vi "TSM Digital Close Sessions.vi"(0 "TSM context":T1) -> (15 "error out":errorcluster)   [LabVIEW 2019]
doc: "Use this VI to reset and close all sessions for all NI-Digital Pattern instruments in the Semiconductor Module Context."
uses:
  <vilib>/NI_TestStand_SemiconductorModule/NI_TestStand_Semiconductor_Module.lvlibp/PinMap/General/SemiconductorModuleContext.ctl
  <vilib>/NI_TestStand_SemiconductorModule/NI_TestStand_Semiconductor_Module.lvlibp
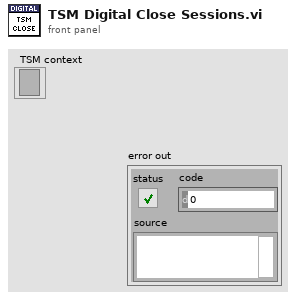
[diagram p1: front panel]
types:
  T1 = typedef "NI_TestStand_Semiconductor_Module.lvlibp/SemiconductorModuleContext.ctl" = refnum<k7>
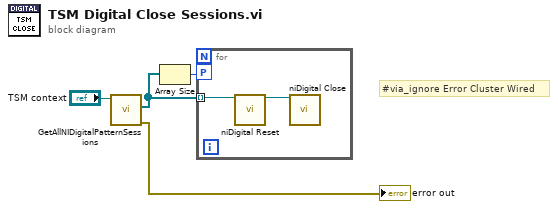
[diagram p0: block diagram]
diagram:
  # "#via_ignore Error Cluster Wired"
  n1 = call <vilib>:"GetAllNIDigitalPatternSessions.vi"("Semiconductor Module Context"="TSM context") -> ("error out"=→"error out":errorcluster, "Instrument Sessions"=w2:refnum<k15>[])  [unwired: 8 in, 1 out]
  n2 = Array Size(array=w2) -> (size(s)=w3:i32)
  n3 = for {
    tunnel: w2 -> [w6] mode=indexing
    workers-P: w3 -> [_]
    n4 = call <instrlib>:"niDigital Reset.vi"("instrument handle in"=w6) -> ("instrument handle out"=w5:refnum<k15>)  [unwired: 13 in, 1 out]
    n5 = call <instrlib>:"niDigital Close.vi"("instrument handle"=w5) -> ()  [unwired: 14 in, 1 out]
  }
